vi "Read User & Password.vi"(8 "error in (no error)":errorcluster, 11 "Path":path) -> (0 "error out":errorcluster, 3 "Array":cluster{"value":string, "value":string, i32}[](array[cluster]))   [LabVIEW 2014]
uses:
  <vilib>/Utility/config.llb/NI_LVConfig.lvlib
  <vilib>/Utility/config.llb/Read Key (String).vi
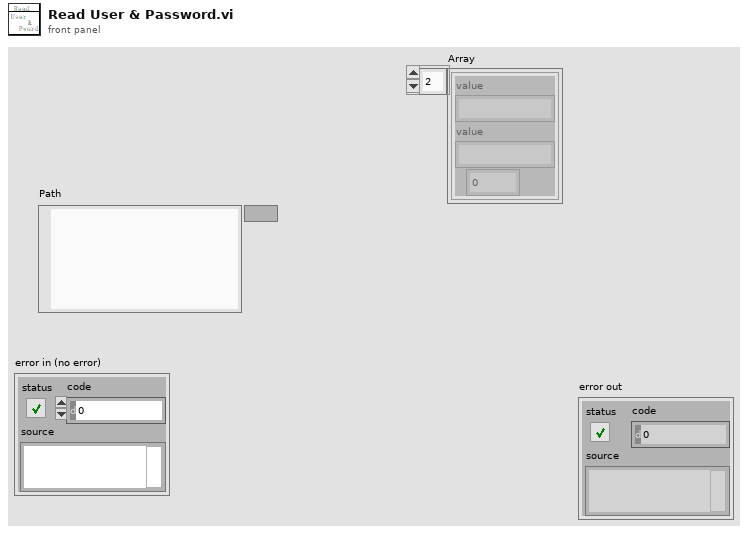
[diagram p1: front panel]
types:
  T1 = typedef "NI_LVConfig.lvlib/Config Data RefNum.ctl" = refnum<k1>
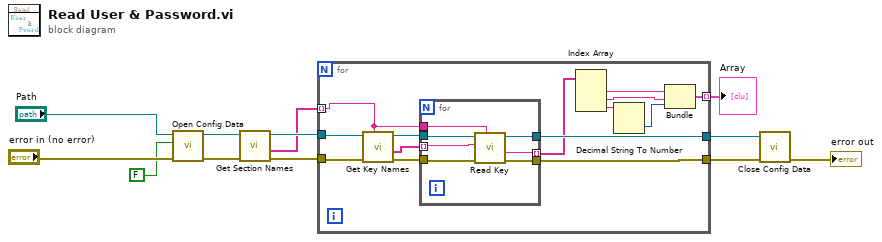
[diagram p0: block diagram]
diagram:
  n1 = call <vilib>:"Open Config Data.vi"("error in (no error)"="error in (no error)", "create file if necessary (T)"=FALSE, "configuration file path"="Path") -> ("error out"=w9:errorcluster, "refnum"=w8:T1)  [unwired: 6 in, 1 out]
  n2 = call <vilib>:"Get Section Names.vi"("error in (no error)"=w9, "refnum"=w8) -> ("error out"=w7:errorcluster, "section names"=w5:string[], "refnum out"=w6:T1)  [unwired: 7 in]
  n3 = for {
    tunnel: w7 -> [w26]
    tunnel: w6 -> [w25]
    tunnel: w5 -> [w22] mode=indexing
    tunnel: [w20] -> w3
    tunnel: [w19] -> w4
    tunnel: [w13] -> w1 mode=indexing
    n4 = call <vilib>:"Get Key Names.vi"("section"=w22, "error in (no error)"=w26, "refnum"=w25) -> ("error out"=w24:errorcluster, "key names"=w21:string[], "refnum out"=w23:T1)  [unwired: 5 in, 1 out]
    n5 = for {
      tunnel: w24 -> [w33]
      tunnel: w23 -> [w32]
      tunnel: w22 -> [w31]
      tunnel: w21 -> [w30] mode=indexing
      tunnel: [w29] -> w20
      tunnel: [w28] -> w18 mode=indexing
      tunnel: [w27] -> w19
      n6 = call-poly <vilib>:"Read Key.vi"("section"=w31, "error in (no error)"=w33, "key"=w30, "refnum"=w32) -> ("error out"=w27:errorcluster, "value"=w28:string, "refnum out"=w29:T1)  [unwired: 4 in, 1 out]
    }
    n7 = Index Array(array=w18) -> (element #1=w16:string, element #2=w15:string, element #3=w17:string)  [unwired: 3 in]
    n8 = Decimal String To Number(string=w17) -> (number=w14:i32)  [unwired: 2 in, 1 out]
    n9 = Bundle("value"=w16, "value"=w15, w14) -> (w13:cluster{"value":string, "value":string, i32})  [unwired: 1 in]
  }
  "Array" <- w1
  n10 = call <vilib>:"Close Config Data.vi"("error in (no error)"=w4, "refnum"=w3) -> ("error out"=→"error out":errorcluster)  [unwired: 8 in, 1 out]
